vi "Write Door Buttons.vi"(8 "error in (no error)":errorcluster, 10 "Door Buttons":T1, 11 "User Console in":refnum<class "User Console.lvclass">) -> (0 "error out":errorcluster, 3 "User Console out":refnum<class "User Console.lvclass">)   [LabVIEW 2019, in "User Console Actor.lvlib" / "User Console.lvclass"]
uses:
  User Console.lvclass
  Door Buttons.ctl
  User Console.lvclass/User Console.ctl
  Abstract User Console Actor/Abstract User Console Actor/Abstract User Console.lvclass
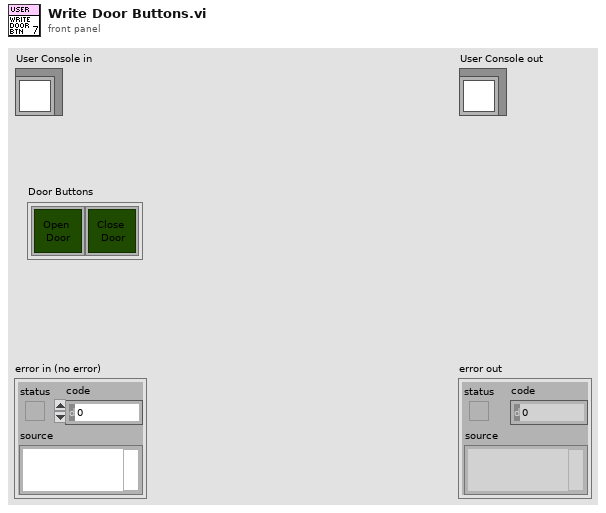
[diagram p1: front panel]
types:
  T1 = typedef "User Console Actor.lvlib/User Console.lvclass/Door Buttons.ctl" = cluster{"Open Door":bool, "Close Door":bool}
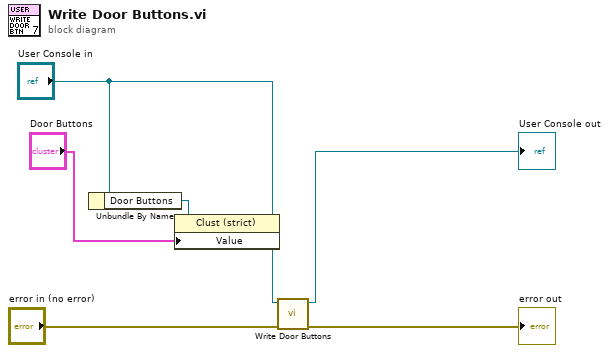
[diagram p0: block diagram]
diagram:
  n1 = Unbundle By Name("User Console in") -> ("Door Buttons"=w2:refnum<vi>)
  n2 = property class="Clust (strict)"(reference=w2, "Value"="Door Buttons") -> ()  [unwired: 1 in, 2 out]
  n3 = call-parent "Write Door Buttons.vi"("error in (no error)"="error in (no error)", "Abstract User Console in"="User Console in") -> ("error out"=→"error out":errorcluster, "Abstract User Console out"=→"User Console out":refnum<class "User Console.lvclass">)  [unwired: 8 in]
